vi "S8300E_GetUUTMAC_EyeChk_WIH.vi"() -> ()   [LabVIEW 2011]
panel:
  out "UUT MAC List":string
  out "CMD-LIST":cluster{string, string, string, string}[](array[cluster])
  out "log msg":string
  out "VISA resource name out":refnum<visa-resource-name>
  out "BEGIN TIME":u32
  out "進行狀況":string
  # "2015-6-1"
  # "Error Code:MAC-PORT1\nError Code:MAC-PORT2\nError Code:MAC-PORT3"
  # "S8300E UUT 3 Ports MAC (接UART COM9)"
  # "目檢待測物 MAC Address"
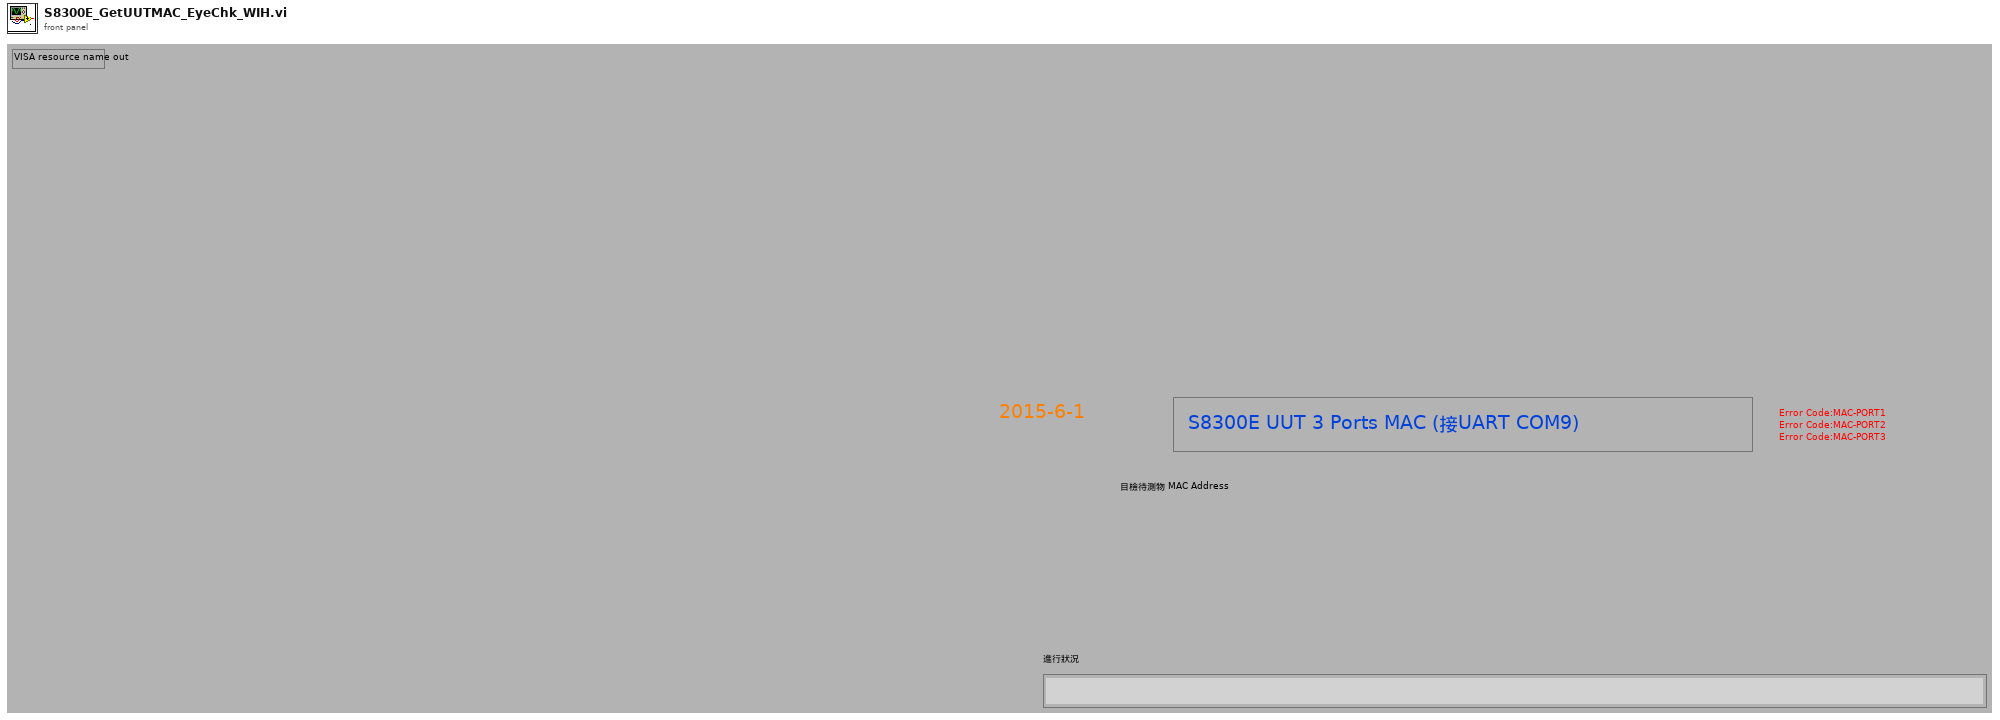
[diagram p1: front panel]
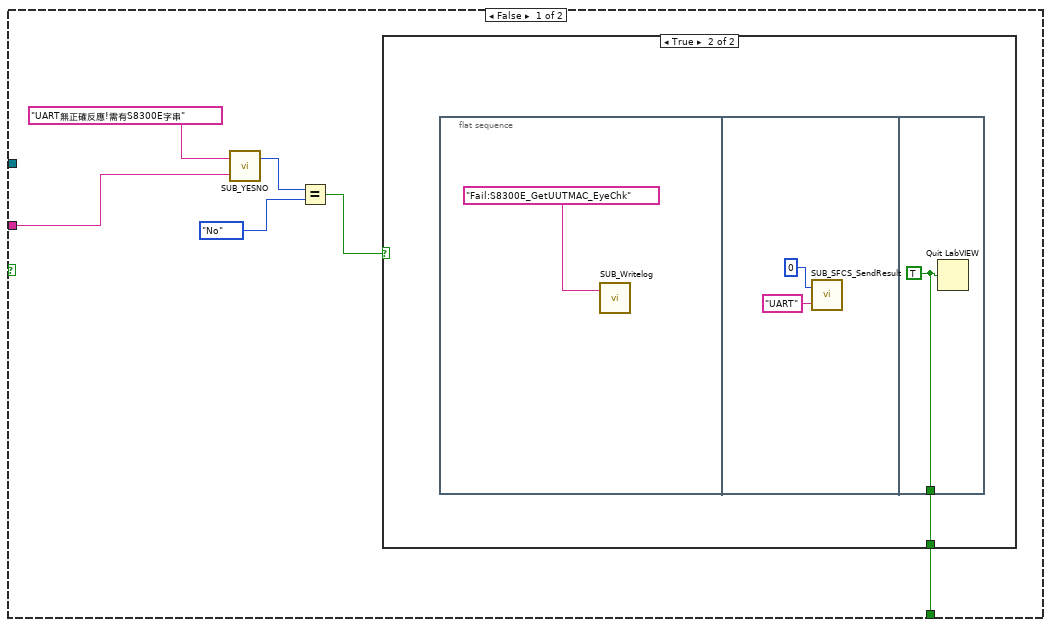
[diagram p5: hidden frame]
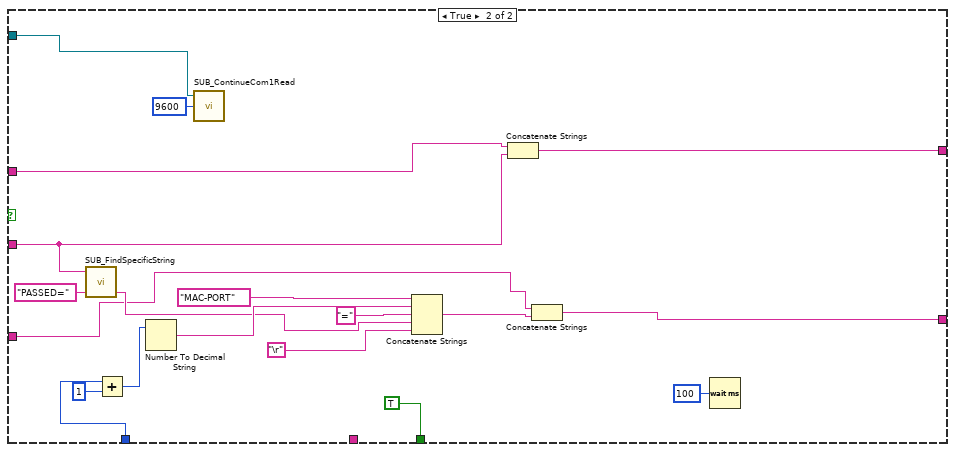
[diagram p8: hidden frame]
diagram:
  n1 = flat-sequence {
    frame #0 {
      n2 = Tick Count (ms)() -> (millisecond timer value=→"BEGIN TIME":u32)
    }
    frame #1 {
      n3 = property on="進行狀況" class="Str"("Blinking"=TRUE) -> ()  [unwired: 2 in, 2 out]
      "進行狀況" <- "進入測試準備中...." ("進行狀況")
    }
    frame #2 {
      n4 = call "SUB_SearchFile_inFolder.vi"("Search Filename in Folder"="S8300E_sfcs_misc.txt") -> ("File Existing True/Flase"=w4:bool)  [unwired: 1 in]
      n5 = case shown="False" w4 {
        frame False {
          n6 = flat-sequence {
            frame #0 {
              n7 = call "Display Message to User"() -> ()  [unwired: 10 in, 2 out]
            }
            frame #1 {
              n8 = call "SUB_Writelog.vi"("Pass/Fail"="Fail:S8300E_GetUUTMAC_EyeChk") -> ()  [unwired: 2 in]
            }
            frame #2 {
              n9 = Quit LabVIEW(quit? (T)=TRUE) -> ()
            }
          }
        }
        frame True {
        }
      }
    }
    frame #3 {
      n10 = Concatenate Strings("./mac.sh -r -e  1", "\r") -> (w28:string)
      n11 = Concatenate Strings("./mac.sh -r -e  2", "\r") -> (w24:string)
      n12 = Concatenate Strings("./mac.sh -r -e  3", "\r") -> (w20:string)
      n13 = Bundle(w28, ";", "Checking MAC-PORT1..", "MAC-PORT1") -> (w14:cluster{string, string, string, string})  [unwired: 1 in]
      n14 = Bundle(w24, ";", "Checking MAC-PORT2...", "MAC-PORT2") -> (w13:cluster{string, string, string, string})  [unwired: 1 in]
      n15 = Bundle(w20, ";", "Checking MAC-PORT3...", "MAC-PORT3") -> (w12:cluster{string, string, string, string})  [unwired: 1 in]
      n16 = Build Array(w14, w13, w12) -> (→"CMD-LIST":cluster{string, string, string, string}[])
    }
    frame #4 {
      n17 = call "SUB_COM1_CLOSE.vi"("VISA resource name"=refnum<visa-resource-name> "COM9") -> ()  [unwired: 3 in]
    }
    frame #5 {
      n18 = case shown="True" TRUE {
        frame False {
        }
        frame True {
          n19 = call "SUB_COM9_INIT.vi"("baud rate"=u32 115200) -> ("VISA resource name out"=w35:refnum<visa-resource-name>)  [unwired: 1 in, 1 out]
          "VISA resource name out" <- w35
          n20 = call "SUB_COM1Wrt.vi"("VISA resource name"=w35, "write buffer"="\r") -> ("duplicate VISA resource name"=w32:refnum<visa-resource-name>)  [unwired: 1 in, 1 out]
          n21 = call "SUB_ContinueCom1Read.vi"("Numeric"=9600, "duplicate VISA resource name 2"=w32) -> ()  [unwired: 1 in, 3 out]
        }
      }
    }
    frame #6 {
      n22 = case shown="True" TRUE {
        frame False {
        }
        frame True {
          n23 = while {
            stop <- w45 stop-if-true
            n24 = local read "VISA resource name out"() -> (w39:refnum<visa-resource-name>)
            n25 = call "SUB_COM1Wrt.vi"("VISA resource name"=w39, "write buffer"="\r") -> ("duplicate VISA resource name"=w38:refnum<visa-resource-name>)  [unwired: 1 in, 1 out]
            n26 = Tick Count (ms)() -> (millisecond timer value=w44:u32)
            n27 = call "SUB_READ_COM1_FindString_timeout.vi"("Find this String"="s8300e_func_test#", "Timeout Seccond"=3.0, "Begin time"=w44, "duplicate VISA resource name 2"=w38) -> ("Output String"=w40:string, "Found String"=w41:bool)  [unwired: 1 in, 1 out]
            n28 = case shown="True" w41 {
              tunnel: [w48 TRUE] -> w45
              tunnel: w40 -> [w47 _]
              tunnel: w38 -> [_ w58]
              frame False {
                n29 = call "SUB_YESNO.vi"("Debug View"=w47, "Status"="UART無正確反應!需有S8300E字串") -> ("yes/no"=w51:enum32{"No Selection", "Yes", "No", "None"})  [unwired: 1 in]
                n30 = Equal?(x=w51, y=enum32{"No Selection", "Yes", "No", "None"}."No") -> (x = y?=w49:bool)
                n31 = case shown="True" w49 {
                  tunnel: [_ w53] -> w48
                  frame False {
                  }
                  frame True {
                    n32 = flat-sequence {
                      tunnel: [w57] -> w53
                      frame #0 {
                        n33 = call "SUB_Writelog.vi"("Pass/Fail"="Fail:S8300E_GetUUTMAC_EyeChk") -> ()  [unwired: 2 in]
                      }
                      frame #1 {
                        n34 = call "SUB_SFCS_SendResult.vi"("ErrorCode"="UART", "PASS_Fail (1/0)"=i8 0) -> ()  [unwired: 1 out]
                      }
                      frame #2 {
                        w57 = TRUE ("quit? (T)")
                        n35 = Quit LabVIEW(quit? (T)=w57) -> ()
                      }
                    }
                  }
                }
              }
              frame True {
                n36 = call "SUB_ContinueCom1Read.vi"("Numeric"=9600, "duplicate VISA resource name 2"=w58) -> ()  [unwired: 1 in, 3 out]
              }
            }
          }
        }
      }
    }
    frame #7 {
      n37 = local read "CMD-LIST"() -> (w63:cluster{string, string, string, string}[])
      n38 = Array Size(array=w63) -> (size(s)=w66:i32)
      n39 = for {
        N: w66 -> [_]
        shift-right: [w71] -> w64
        shift-left: "" -> [w70]
        shift-right: [w68] -> w61
        shift-left: "" -> [w67]
        i -> [w69]
        n40 = while {
          tunnel: w69 -> [w93]
          tunnel: [w88] -> w71
          tunnel: w70 -> [w87]
          tunnel: w69 -> [w80]
          tunnel: [w79] -> w68
          tunnel: w67 -> [w78]
          stop <- w89 stop-if-true
          n41 = local read "CMD-LIST"() -> (w86:cluster{string, string, string, string}[])
          n42 = local read "VISA resource name out"() -> (w72:refnum<visa-resource-name>)
          n43 = Index Array(array=w86, index=w93) -> (element=w85:cluster{string, string, string, string})
          n44 = call "SUB_ContinueCom1Read.vi"("Numeric"=9600, "duplicate VISA resource name 2"=w72) -> ("duplicate VISA resource name"=w73:refnum<visa-resource-name>)  [unwired: 1 in, 2 out]
          n45 = Unbundle(w85) -> (w84:string, w82:string, w83:string, w81:string)
          n46 = call "SUB_COM1Wrt.vi"("VISA resource name"=w73, "write buffer"=w84) -> ("duplicate VISA resource name"=w92:refnum<visa-resource-name>)  [unwired: 1 in, 1 out]
          n47 = Tick Count (ms)() -> (millisecond timer value=w91:u32)
          n48 = call "SUB_READ_COM1_FindString_timeout.vi"("Find this String"=w82, "Timeout Seccond"=5.0, "Begin time"=w91, "duplicate VISA resource name 2"=w92) -> ("Output String"=w77:string)  [unwired: 1 in, 2 out]
          n49 = local write "進行狀況"(w83) -> ()
          n50 = call "SUB_FindSpecificString.vi"("Find this String"="PASSED=", "String data"=w77) -> ("Found"=w75:bool)  [unwired: 2 in, 1 out]
          n51 = case shown="False" w75 {
            tunnel: [_ TRUE] -> w89
            tunnel: w77 -> [w104 w124]
            tunnel: [w100 w129] -> w88
            tunnel: w87 -> [w100 w128]
            tunnel: w81 -> [w99 _]
            tunnel: w80 -> [_ w120]
            tunnel: [w94 w116] -> w79
            tunnel: w78 -> [w94 w115]
            tunnel: w72 -> [_ w112]
            frame False {
              n52 = local read "進行狀況"() -> (w96:string)
              n53 = Concatenate Strings("USB測試失敗!有接U盤?" ("string"), "\r", w96) -> (w95:string)
              n54 = call "SUB_YESNO.vi"("Debug View"=w104, "Status"=w95) -> ("yes/no"=w103:enum32{"No Selection", "Yes", "No", "None"})  [unwired: 1 in]
              n55 = Equal?(x=w103, y=enum32{"No Selection", "Yes", "No", "None"}."No") -> (x = y?=w101:bool)
              n56 = case shown="True" w101 {
                tunnel: w99 -> [_ w105]
                frame False {
                }
                frame True {
                  n57 = flat-sequence {
                    tunnel: [w107] -> w106
                    tunnel: w105 -> [w107]
                    tunnel: w106 -> [w109]
                    frame #0 {
                      n58 = call "SUB_Writelog.vi"("Pass/Fail"="Fail:S8300E_GetUUTMAC_EyeChk") -> ()  [unwired: 2 in]
                    }
                    frame #1 {
                      n59 = call "SUB_SFCS_SendResult.vi"("ErrorCode"=w109, "PASS_Fail (1/0)"=i8 0) -> ()  [unwired: 1 out]
                    }
                    frame #2 {
                      n60 = Quit LabVIEW(quit? (T)=TRUE) -> ()
                    }
                  }
                }
              }
            }
            frame True {
              n61 = call "SUB_FindSpecificString.vi"("Find this String"="PASSED=", "String data"=w124) -> ("before \"; \" string"=w122:string)  [unwired: 2 in, 1 out]
              n62 = Add(x=w120, y=1) -> (x+y=w118:i32)
              n63 = Number To Decimal String(number=w118) -> (decimal integer string=w126:string)  [unwired: 1 in]
              n64 = call "SUB_ContinueCom1Read.vi"("Numeric"=9600, "duplicate VISA resource name 2"=w112) -> ()  [unwired: 1 in, 3 out]
              n65 = Concatenate Strings("MAC-PORT" ("string"), w126, "=" ("string"), w122, "\r") -> (w117:string)
              n66 = Concatenate Strings(w128, w124) -> (w129:string)
              n67 = Concatenate Strings(w115, w117) -> (w116:string)
              n68 = Wait (ms)(milliseconds to wait=u32 100) -> ()  [unwired: 1 out]
            }
          }
        }
      }
      "log msg" <- w64
      "UUT MAC List" <- w61
    }
    frame #8 {
      n69 = local read "UUT MAC List"() -> (w135:string)
      n70 = Concatenate Strings("請回答如下問題." ("Question:"), "\r", w135) -> (w134:string)
      n71 = call "SUB_ASK_YESNO.vi"("Question:"=w134) -> ("yes/no"=w133:enum32{"No Selection", "Yes", "No", "None"})  [unwired: 2 in]
      n72 = Equal?(x=w133, y=enum32{"No Selection", "Yes", "No", "None"}."No") -> (x = y?=w131:bool)
      n73 = case shown="True" w131 {
        frame False {
        }
        frame True {
          n74 = flat-sequence {
            frame #0 {
              n75 = call "SUB_Writelog.vi"("Pass/Fail"="Fail:S8300E_GetUUTMAC_EyeChk") -> ()  [unwired: 2 in]
            }
            frame #1 {
              n76 = Quit LabVIEW(quit? (T)=TRUE) -> ()
            }
          }
        }
      }
    }
    frame #9 {
      n77 = call "SUB_COM1_CLOSE.vi"("VISA resource name"=refnum<visa-resource-name> "COM9") -> ()  [unwired: 3 in]
    }
    frame #10 {
      w143 = "***Not Good ***" ("replace string (\"\")")
      n78 = local read "log msg"() -> (w147:string)
      n79 = local read "BEGIN TIME"() -> (w152:u32)
      n80 = Tick Count (ms)() -> (millisecond timer value=w151:u32)
      n81 = call "SUB_CAL_TESTTIME.vi"("Test Item name"="S8300E_GetUUTMAC_EyeChk", "Stop tick time"=w151, "Start tick time"=w152) -> ("Test Time output"=w149:string)  [unwired: 2 in]
      n82 = Concatenate Strings("Pass:S8300E_GetUUTMAC_EyeChk", "\n", w147, w149) -> (w142:string)
      n83 = call "SUB_SEARCH_REPLACE_STR.vi"("replace string (\"\")"=w143, "search string"="FAILED", "input string"=w142) -> ("result string"=w145:string)  [unwired: 2 in]
      n84 = call "SUB_SEARCH_REPLACE_STR.vi"("replace string (\"\")"=w143, "search string"="FAIL", "input string"=w145) -> ("result string"=w141:string)  [unwired: 2 in]
      n85 = call "SUB_Writelog.vi"("Pass/Fail"=w141) -> ()  [unwired: 2 in]
    }
    frame #11 {
      n86 = Request Deallocation(TRUE ("flag")) -> ()
    }
    frame #12 {
      n87 = Quit LabVIEW(quit? (T)=TRUE ("stop? (T)")) -> ()
    }
  }
